vi "Read Voltage.vi"(4 "error in (no error)":errorcluster) -> (0 "error out":errorcluster, 3 "voltage":dbl format="%.2f")   [LabVIEW 2014]
doc: "This VI is used in the LabVIEW Core I course.\n\nThis VI simulates taking voltage readings from a DAQ board. Use this VI to replace the DAQ Assistant Express VI in any temperature reading exercises in this course. This VI is used as a subVI in all (Demo) exercises."
panel:
  in  "Readings":dbl[](array[numeric])=[163.0, 163.0, 163.0, 163.0, 163.0, 163.0, 165.0, 169.0, 172.0, 173.0, 172.0, 172.0, 171.0, 171.0, 174.0, 176.0, 177.0, 178.0, 178.0, 179.0, 178.0, 177.0, 176.0, 175.0, 175.0, 174.0, 173.0, 172.0, 172.0, 172.0, 172.0, 172.0, 171.0, 171.0, 170.0, 170.0, 170.0, 172.0, 173.0, 174.0, 175.0, 177.0, 178.0, 178.0, 178.0, 177.0, 176.0, 175.0, 176.0, 178.0, 179.0, 180.0, 179.0, 178.0, 178.0, 176.0, 176.0, 176.0, 174.0, 174.0, 174.0, 173.0, 173.0, 175.0, 176.0, 178.0, 178.0, 177.0, 176.0, 175.0, 175.0, 174.0, 174.0, 173.0, 173.0, 172.0, 172.0, 171.0, 171.0, 170.0, 170.0, 170.0, 170.0, 170.0, 170.0, 170.0, 169.0, 166.0, 167.0, 169.0, 170.0, 169.0, 168.0, 168.0, 168.0, 168.0, 167.0, 167.0, 167.0, 167.0] format="%.2f"
  # "*This VI is a demo version of a \nVI that reads the voltage on\nDevice 1, channel 0 and scales\nthe signal by 100 to convert to\ntemperature.*"
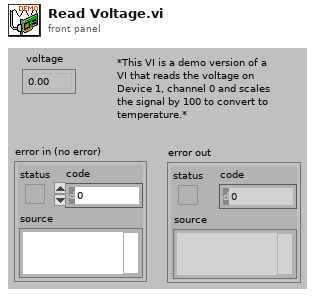
[diagram p1: front panel]
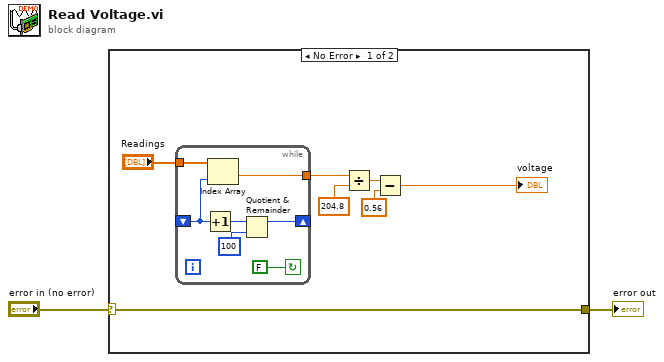
[diagram p0: block diagram]
diagram:
  n1 = case shown="No Error" "error in (no error)" {
    selector: "error in (no error)" -> [w4 w17]
    tunnel: [w4 w17] -> w1
    frame No Error {
      n2 = while {
        tunnel: "Readings" -> [w11]
        tunnel: [w12] -> w7
        shift-left: _ -> [w16]
        shift-right: [w13] -> _
        stop <- FALSE continue-if-true
        n3 = Increment(x=w16) -> (x+1=w15:i32)
        n4 = Index Array(array=w11, index=w16) -> (element=w12:dbl)
        n5 = Quotient & Remainder(x=w15, y=100) -> (x-y*floor(x/y)=w13:i32)  [unwired: 1 out]
      }
      n6 = Divide(x=w7, y=204.8) -> (x/y=w6:dbl)
      n7 = Subtract(x=w6, y=0.56) -> (x-y=→"voltage":dbl)
    }
    frame Error {
    }
  }
  "error out" <- w1
